vi "NavXtoDashBoard.vi"   [LabVIEW 2015]
uses:
  <vilib>/Rock Robotics/Network Tables/NT Write Number.vi
  <instrlib>/navX Library v2/navX Library v2.lvlib
types:
  T1 = typedef "navX Library v2.lvlib/Z900_navX_DeviceTypeDef.ctl" = cluster{"Interface":cluster{"Protocol":T2, "Update Rate (4Hz-60Hz)":u8, "navX Open TypeDef":variant}, "Notify Packet":refnum<notifier>, "Loop VI Refnum":refnum<vi>, "Ready to Close Occurrence Refnum":refnum<k4>}
  T2 = typedef "navX Library v2.lvlib/Z900_navX_ProtocolTypeDef.ctl" = enum16{"SERIAL", "I2C", "SPI"}
  T3 = cluster{"Yaw":dbl, "Roll":dbl, "Pitch":dbl, "Heading":dbl, "Fused Heading":dbl}
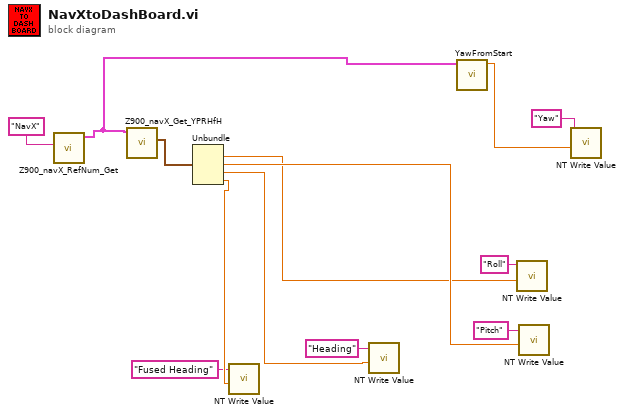
[diagram p0: block diagram]
diagram:
  n1 = call <instrlib>:"Z900_navX_RefNum_Get.vi"("refnum name"="NavX") -> ("navX Device"=w2:T1)  [unwired: 9 in, 1 out]
  n2 = call <instrlib>:"Z900_navX_Get_YPRHfH.vi"("navX Device"=w2) -> ("YRPHfH"=w3:T3)  [unwired: 7 in, 3 out]
  n3 = Unbundle(w3) -> ("Roll"=w5:dbl, "Pitch"=w6:dbl, "Heading"=w11:dbl, "Fused Heading"=w13:dbl)  [unwired: 1 out]
  n4 = call-poly <vilib>:"NT Write Value.vi"("Numeric"=w13, "Name"="Fused Heading") -> ()  [unwired: 9 in, 1 out]
  n5 = call-poly <vilib>:"NT Write Value.vi"("Numeric"=w11, "Name"="Heading") -> ()  [unwired: 9 in, 1 out]
  n6 = call "YawFromStart.vi"("navX Device"=w2) -> ("Yaw"=w4:dbl)  [unwired: 10 in]
  n7 = call-poly <vilib>:"NT Write Value.vi"("Numeric"=w5, "Name"="Roll") -> ()  [unwired: 9 in, 1 out]
  n8 = call-poly <vilib>:"NT Write Value.vi"("Numeric"=w6, "Name"="Pitch") -> ()  [unwired: 9 in, 1 out]
  n9 = call-poly <vilib>:"NT Write Value.vi"("Numeric"=w4, "Name"="Yaw") -> ()  [unwired: 9 in, 1 out]
